vi "TellSelf.vi"(10 "Message":refnum<class "Message.lvclass">, 11 "Actor":refnum<class "Actor.lvclass">) -> (3 "Actor":refnum<class "Actor.lvclass">)   [LabVIEW 2020, in "jettl.lvlib"]
uses:
  jettl.lvlib
  TellOrigin.ctl
  Actor/Actor.lvclass
  Message/Message.lvclass
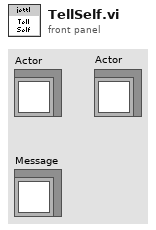
[diagram p1: front panel]
types:
  T1 = typedef "jettl.lvlib/TellOrigin.ctl" = enum16{"Self", "Mediator", "Component"}
  T2 = typedef "jettl.lvlib/Base.ctl" = cluster{"Lifetime":T3, "SelfActor":T4, "MediatorActor":T4, "ComponentActorMap":T9}
  T3 = typedef "jettl.lvlib/Lifetime.ctl" = enum16{"Init", "Spawn", "Setup", "TeardownBeforeRunning", "Running", "StopCalled", "StoppingWithComponents", "StoppingNoComponents", "TeardownAfterRunning", "Stopped"}
  T4 = typedef "jettl.lvlib/Actor.ctl" = cluster{"Messages":T5, "ActorAlias":string, "ActorType":T8, "Transport":refnum<user-event>, "VIRef":refnum<vi>}
  T5 = typedef "jettl.lvlib/Messages.ctl" = cluster{"Listen":T6, "TellSelf":T6, "TellMediator":T6, "TellComponentMap":T7}
  T6 = typedef "jettl.lvlib/MessageSet.ctl" = set{refnum<class "Message.lvclass">}
  T7 = typedef "jettl.lvlib/TellComponentMap.ctl" = map{string, T6}
  T8 = typedef "jettl.lvlib/ActorType.ctl" = enum16{"Mediator", "Component"}
  T9 = typedef "jettl.lvlib/ComponentActorMap.ctl" = map{string, T4}
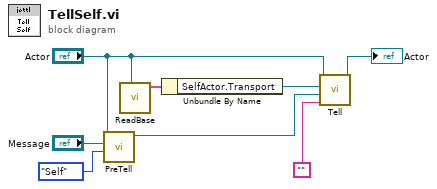
[diagram p0: block diagram]
diagram:
  n1 = call "PreTell.vi"("TellOrigin"=TellOrigin."Self", "Message"="Message", "Actor"="Actor") -> ("Message"=w1:refnum<class "Message.lvclass">)  [unwired: 8 in]
  n2 = call-dynamic "ReadBase.vi"("Actor"="Actor") -> ("BaseActor"=w4:T2)  [unwired: 10 in]
  n3 = Unbundle By Name(w4) -> ("SelfActor.Transport"=w2:refnum<user-event>)
  n4 = call "Tell.vi"("ActorAlias"="", "Message"=w1, "Transport"=w2, "Actor"="Actor") -> ("Actor"=→"Actor":refnum<class "Actor.lvclass">)  [unwired: 7 in]
